vi "SpawnMediator.vi"(8 "Components":T1[](array[typedef]), 9 "Persistent":T1[](array[typedef]), 10 "MediatorAlias":string, 11 "Mediator":refnum<class "Actor.lvclass">) -> ()   [LabVIEW 2020, in "jettl.lvlib"]
uses:
  jettl.lvlib
  Message/Message.lvclass
  Base/Actor/Actor.lvclass
  C:/jettl-harness/repos/jettl/src/jettl/jettl/Base/Actor/Actor.lvclass
  C:/jettl-harness/repos/jettl/src/jettl/jettl/Actor/Actor.lvclass
  Actor/Actor.lvclass
  LifecycleEnum.ctl
  MessageCluster.ctl
  ActorTypeEnum.ctl
  MessageSet.ctl
  TellComponentMessageSetMap.ctl
  MessagesCluster.ctl
  ActorCluster.ctl
  PostSetupCluster.ctl
  SpawnComponent.vi
  MainCluster.ctl
  Base/Base.lvlib
  TellOriginEnum.ctl
  MetadataCluster.ctl
  ActorMap.ctl
  CustomMetadata/CustomMetadata.lvclass
panel:
  in  "Component":refnum<class "Actor.lvclass">
  in  "Actor in 2":refnum<class "Actor.lvclass">
  in  "Actors 2":refnum<class "Actor.lvclass">[](array[class])
  out "Actor out 2":refnum<class "Actor.lvclass">
  out "Actor out":refnum<class "Actor.lvclass">
  in  "Actor in":refnum<class "Actor.lvclass">
  in  "Actors":refnum<class "Actor.lvclass">[](array[class])
  in  "ActorAlias":string
  in  "Error in 2":errorcluster
  out "Error out 2":errorcluster
  in  "Teller 2":T2 {"AbsoluteTime" format="%<%x %.3X>T"}
  out "ConcreteActor 4":refnum<class "Actor.lvclass">
  in  "ConcreteActor 3":refnum<class "Actor.lvclass">
  in  "Error in":errorcluster
  out "Error out":errorcluster
  in  "Error":errorcluster
  in  "Teller":T2 {"AbsoluteTime" format="%<%x %.3X>T"}
  in  "Actor 2":refnum<class "Actor.lvclass">
  out "ConcreteActor":refnum<class "Actor.lvclass">
  in  "ConcreteActor 2":refnum<class "Actor.lvclass">
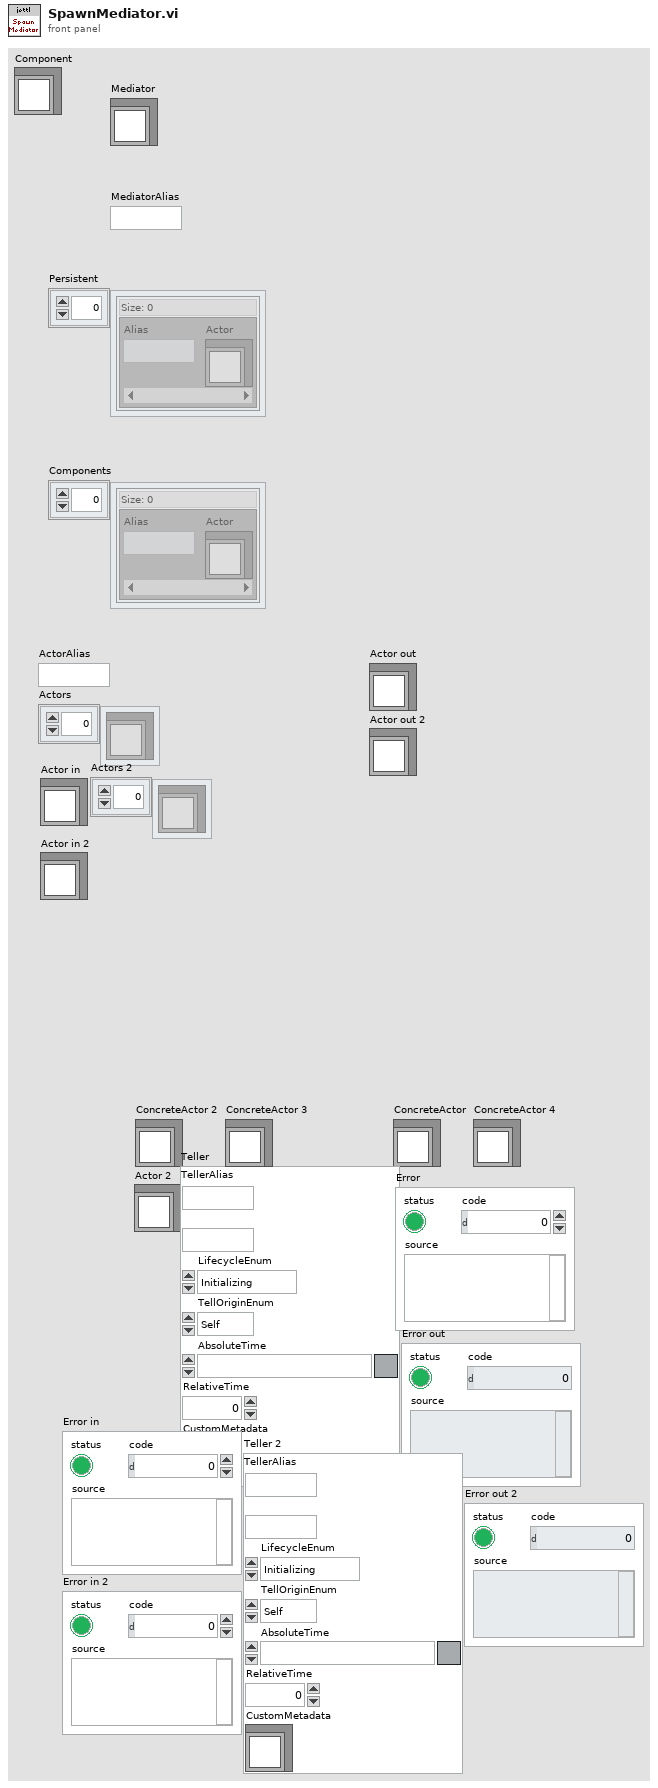
[diagram p1: front panel]
types:
  T1 = typedef "jettl.lvlib/ActorMap.ctl" = map{string, refnum<class "Actor.lvclass">}
  T2 = typedef "jettl.lvlib/MetadataCluster.ctl" = cluster{"TellerAlias":string, "ListenerAlias":string, "LifecycleEnum":T3, "TellOriginEnum":T4, "AbsoluteTime":timestamp, "RelativeTime":dbl, "CustomMetadata":refnum<class "CustomMetadata.lvclass">}
  T3 = typedef "jettl.lvlib/LifecycleEnum.ctl" = enum16{"Initializing", "SettingUp", "Starting", "Running", "Stopping", "TearingDown", "Terminated"}
  T4 = typedef "jettl.lvlib/TellOriginEnum.ctl" = enum16{"Self", "Mediator", "Component"}
  T5 = typedef "jettl.lvlib/MainCluster.ctl" = cluster{"SetupClusterQueue":refnum<queue>, "BeginSetupQueue":refnum<queue>, "SetupErrorQueue":refnum<queue>, "BeginStartQueue":refnum<queue>}
  T6 = typedef "jettl.lvlib/PostSetupCluster.ctl" = cluster{"VIRef":refnum<vi>, "Error":errorcluster}
  T7 = typedef "jettl.lvlib/ActorCluster.ctl" = cluster{"MessagesCluster":T8, "Alias":string, "ActorTypeEnum":T11, "MessageClusterDVREvent":refnum<user-event>, "EventRegistrationRef":refnum<event-registration>, "VIRef":refnum<vi>}
  T8 = typedef "jettl.lvlib/MessagesCluster.ctl" = cluster{"ListenMessageSet":T9, "TellSelfMessageSet":T9, "TellMediatorMessageSet":T9, "TellComponentMessageSetMap":T10}
  T9 = typedef "jettl.lvlib/MessageSet.ctl" = set{refnum<class "Message.lvclass">}
  T10 = typedef "jettl.lvlib/TellComponentMessageSetMap.ctl" = map{string, T9}
  T11 = typedef "jettl.lvlib/ActorTypeEnum.ctl" = enum16{"Mediator", "Component"}
  T12 = typedef "jettl.lvlib/BaseCluster.ctl" = cluster{"LifecycleEnum":T3, "MainCluster":T5, "SelfActorCluster":T7, "MediatorActorCluster":T7, "ComponentActorClusterMap":T13}
  T13 = typedef "jettl.lvlib/ComponentActorClusterMap.ctl" = map{string, T7}
  T14 = typedef "jettl.lvlib/AliasTellComponent.ctl" = map{string, T15}
  T15 = typedef "jettl.lvlib/Actor.ctl" = cluster{"Messages":T16, "ActorAlias":string, "ActorType":T18, "Transport":refnum<user-event>, "EventRegistrationRef":refnum<event-registration>, "VIRef":refnum<vi>}
  T16 = typedef "jettl.lvlib/Messages.ctl" = cluster{"Listen":T9, "TellSelf":T9, "TellMediator":T9, "TellComponentMap":T17}
  T17 = typedef "jettl.lvlib/TellComponent.ctl" = map{string, T9}
  T18 = typedef "jettl.lvlib/ActorType.ctl" = enum16{"Mediator", "Component"}
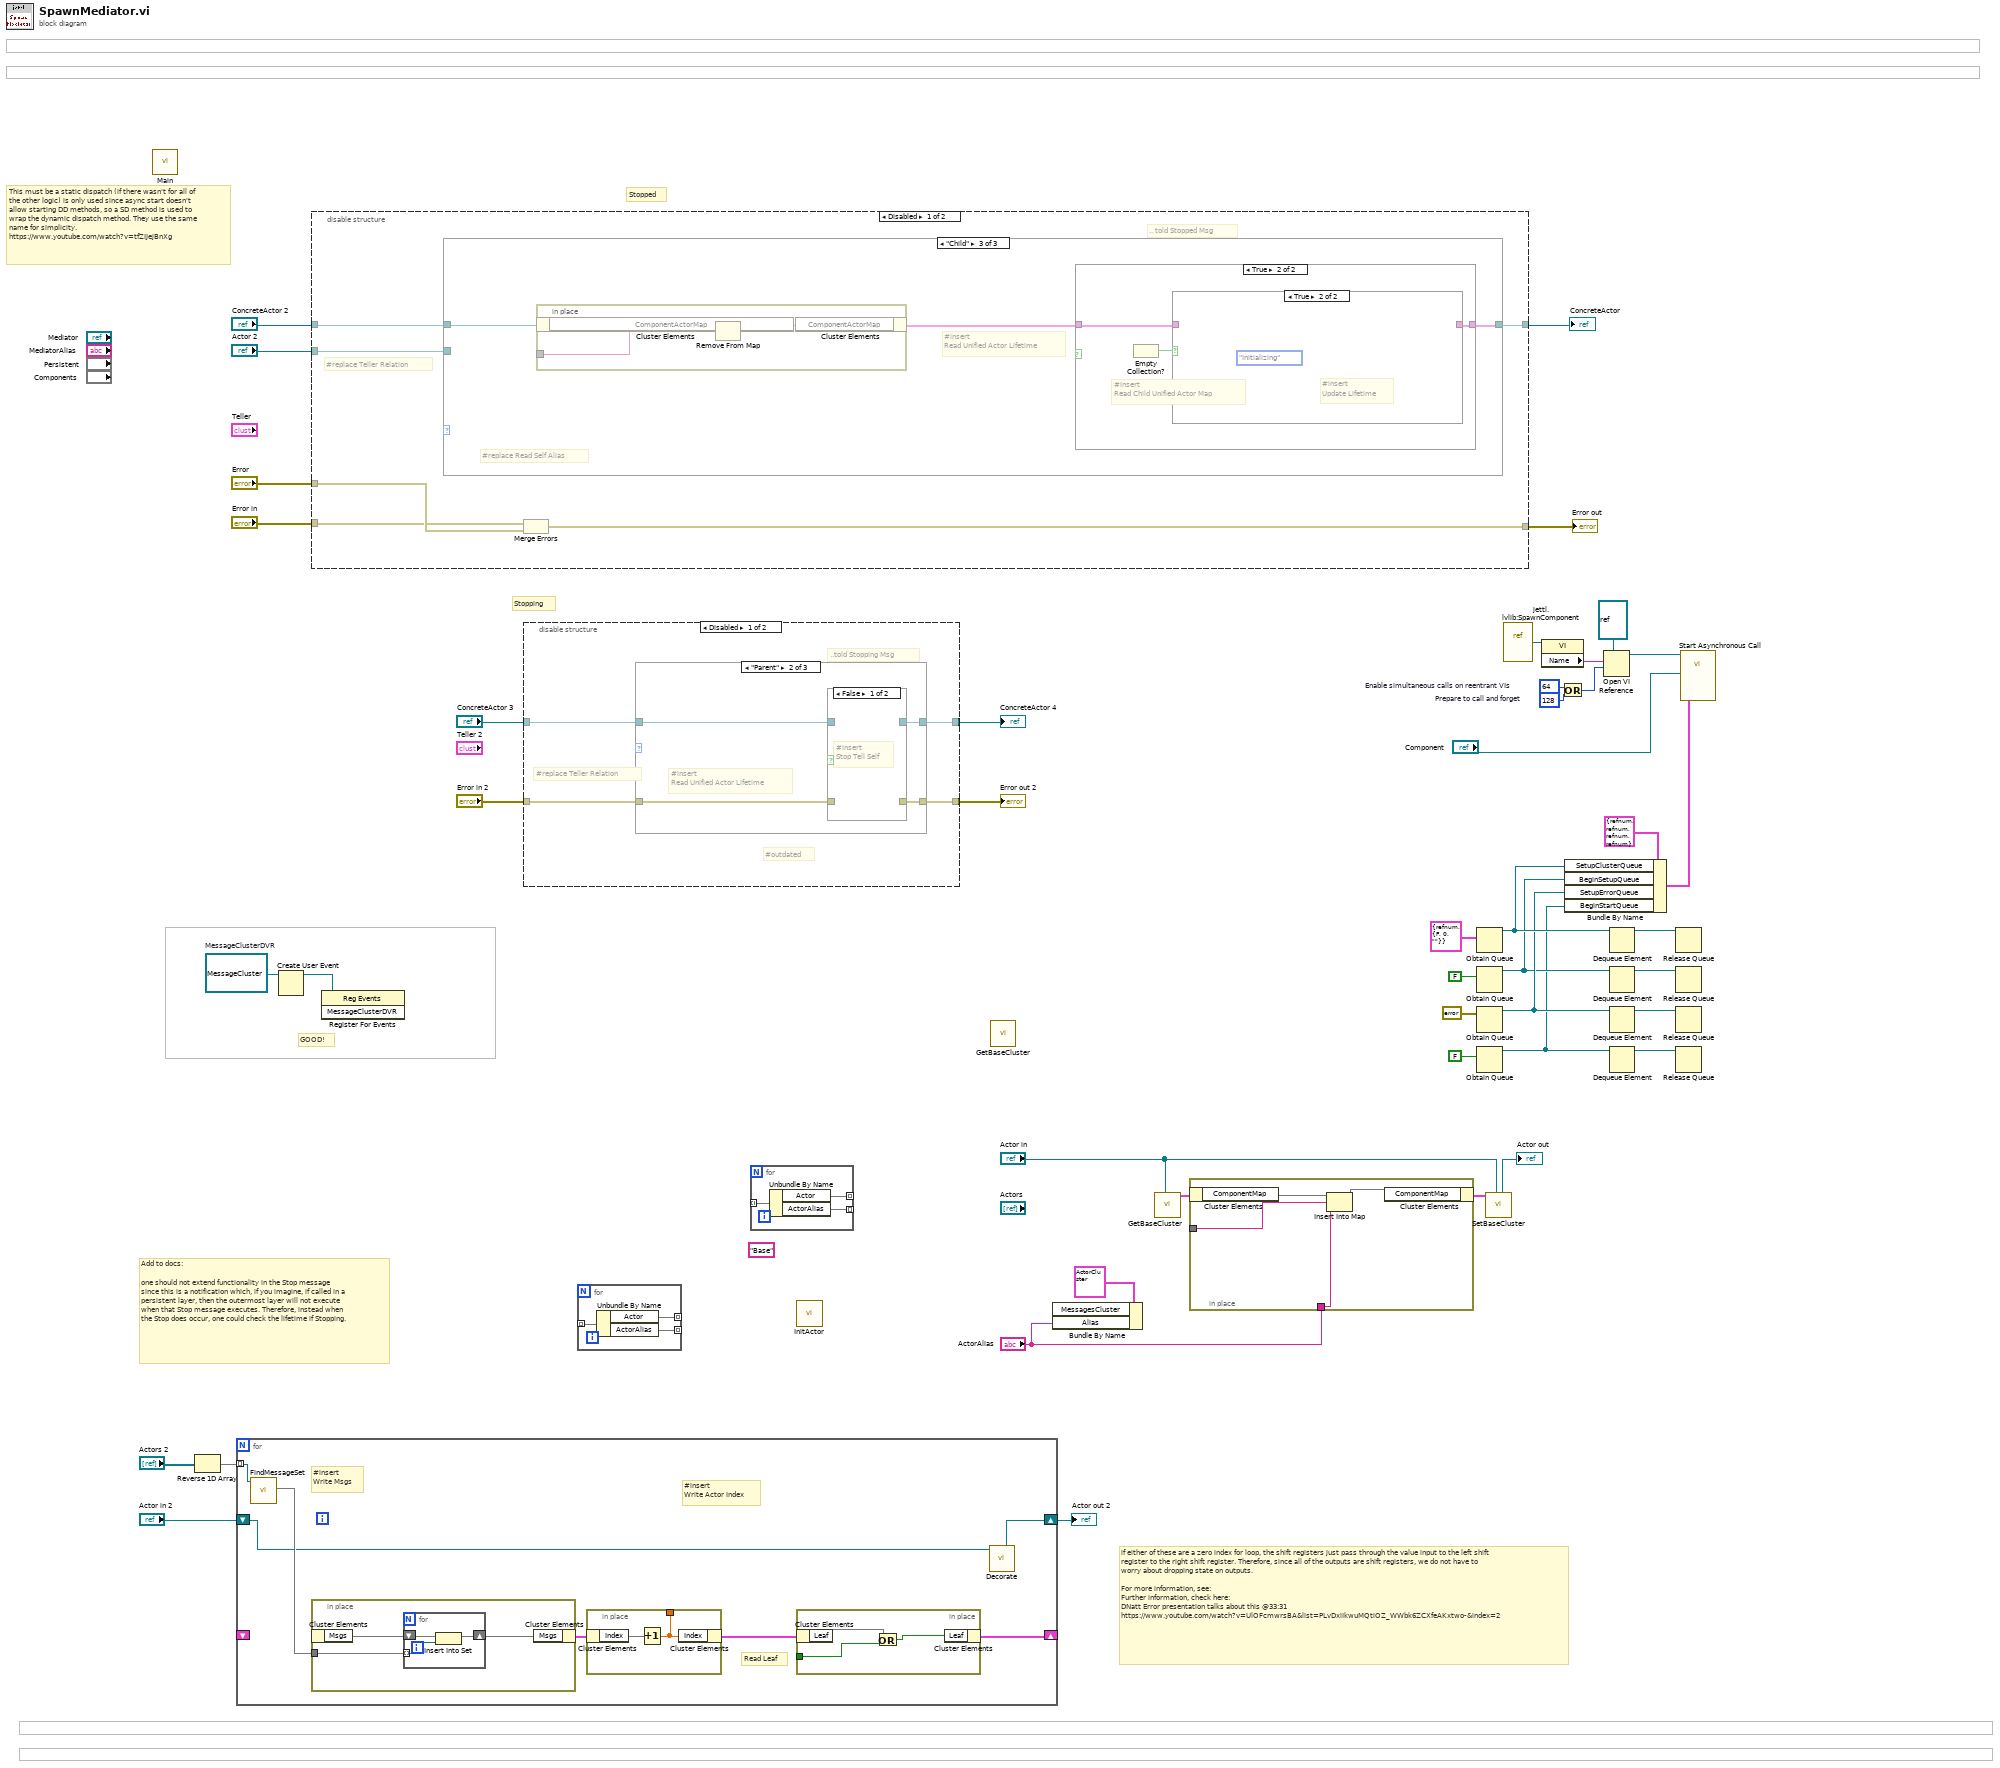
[diagram p0: block diagram]
diagram:
  w3 = refnum<data-value> refnum  # MessageClusterDVR
  w10 = 64  # Enable simultaneous calls on reentrant VIs
  w11 = 128  # Prepare to call and forget
  (unwired) "Base"
  # "GOOD!"
  # "if either of these are a zero index for loop, the shift registers just pass through the value input to the left shift register to the right shift register. Therefore, since all of the outputs are shift registers, we do not have to worry about dropping state on outputs.\n\nFor more information, see:\nFurther information, check here:\nDNatt Error presentation talks about this @33:31\nhttps://www.youtube.com/watch?v=UlOFcmwrsBA&list=PLvDxiIkwuMQtiOZ_WWbk6ZCXfeAKxtwo-&index=2"
  # "Add to docs:\n\none should not extend functionality in the Stop message since this is a notification which, if you imagine, if called in a persistent layer, then the outermost layer will not execute when that Stop message executes. Therefore, instead when the Stop does occur, one could check the lifetime if Stopping."
  # "Stopped"
  # "Stopping"
  # "This must be a static dispatch (if there wasn't for all of the other logic) is only used since async start doesn't allow starting DD methods, so a SD method is used to wrap the dynamic dispatch method. They use the same name for simplicity.\nhttps://www.youtube.com/watch?v=tfZIJejBnXg"
  n1 = call-dynamic "Main.vi"() -> ()  [unwired: 12 in]
  n2 = Reverse 1D Array(array="Actors 2") -> (reversed array=w33:refnum<class "Actor.lvclass">[])
  n3 = for {
    tunnel: w33 -> [w56] mode=indexing
    shift-right: [w51] -> w32
    shift-left: "Actor in 2" -> [w49]
    shift-right: [w57] -> w29
    shift-left: _ -> [_]
    # "#insert\nWrite Actor Index"
    # "#insert\nWrite Msgs"
    # "Read Leaf"
    n4 = call-dynamic "FindMessageSet.vi"(11:w56) -> (2:w58)  [unwired: 9 in, 1 out]
    n5 = in-place {
      in-place-border: w58 -> [w66]
      n6 = in-place-cluster #1() -> ("Msgs"=w65)  [unwired: 1 in]
      n7 = for {
        shift-right: [w68] -> w64
        shift-left: w65 -> [w69]
        tunnel: w66 -> [w67] mode=indexing
        n8 = Insert Into Set(10:w67, 11:w69) -> (3:w68:set{refnum<class "Message.lvclass">})  [unwired: 1 out]
      }
      n9 = in-place-cluster #1("Msgs"=w64) -> (w54:cluster{})
    }
    n10 = in-place {
      in-place-border: [w62] -> w52
      n11 = in-place-cluster #2(w54) -> ("Index"=w63)
      n12 = Increment(x=w63) -> (x+1=w62:dbl)
      n13 = in-place-cluster #2("Index"=w62) -> (w53:cluster{})
    }
    n14 = in-place {
      in-place-border: [w59] -> w55
      n15 = in-place-cluster #3(w53) -> ("Leaf"=w61)
      n16 = Or(x=w61, y=w59) -> (x .or. y?=w60:bool)
      n17 = in-place-cluster #3("Leaf"=w60) -> (w57:cluster{})
    }
    n18 = call-dynamic "Decorate.vi"("Actor"=w49) -> (5:"Actor"=w51:refnum<class "Actor.lvclass">, 7:"Actor"=w50:refnum<class "Actor.lvclass">)  [unwired: 9 in]
  }
  "Actor out 2" <- w32
  n19 = Create User Event(user event datatype=w3) -> (user event=w2:refnum<user-event>)  [unwired: 1 in, 1 out]
  n20 = disable-structure shown="Disabled" {
    disable-tunnel: [w75 w93] -> w48
    disable-tunnel: "ConcreteActor 2" -> [w74 w93]
    disable-tunnel: "Actor 2" -> [w73 _]
    disable-tunnel: "Error" -> [w72 _]
    disable-tunnel: "Error in" -> [w71 w94]
    disable-tunnel: [w70 w94] -> w43
    frame Disabled {
      # "#replace Teller Relation"
      # ".. told Stopped Msg"
      n21 = case shown="\"Child\"" {
        selector: _ -> [_ _ _]
        tunnel: w74 -> [w76 w77 w79]
        tunnel: [w76 w77 w81] -> w75
        tunnel: w73 -> [_ _ w80]
        frame "Self" {
          # "Case will not fundamentally execute"
        }
        frame "Parent" {
          # "Case will not fundamentally execute"
        }
        frame "Child" {
          # "#insert\nRead Unified Actor Lifetime"
          # "#replace Read Self Alias"
          n22 = in-place {
            in-place-border: [w84] -> _
            n23 = in-place-cluster #4(w79) -> ("ComponentActorMap"=w83)
            n24 = Remove From Map(11:w83) -> (3:w82:map{string, i32}, 10:w84:string)  [unwired: 2 out]
            n25 = in-place-cluster #4("ComponentActorMap"=w82) -> (w78:cluster{})
          }
          n26 = case shown="True" {
            selector: _ -> [_ _]
            tunnel: w78 -> [w85 w86]
            tunnel: [w85 w88] -> w81
            frame False {
            }
            frame True {
              # "#insert\nRead Child Unified Actor Map"
              n27 = Empty Collection?() -> (0:w87:bool)  [unwired: 1 in]
              n28 = case shown="True" w87 {
                tunnel: [w89 w90] -> w88
                tunnel: w86 -> [w89 w91]
                frame False {
                }
                frame True {
                  w92 = LifecycleEnum."Initializing" ("Lifetime")
                  # "#insert\nUpdate Lifetime"
                }
              }
            }
          }
        }
      }
      n29 = Merge Errors(w71, w72) -> (w70:errorcluster)
    }
    frame Enabled {
    }
  }
  "ConcreteActor" <- w48
  "Error out" <- w43
  n30 = register-events(w2) -> (reference out=w1:refnum<event-registration>)  [unwired: 2 in, 1 out]
  n31 = disable-structure shown="Disabled" {
    disable-tunnel: "ConcreteActor 3" -> [w98 w113]
    disable-tunnel: [w97 w113] -> w41
    disable-tunnel: "Error in 2" -> [w96 w112]
    disable-tunnel: [w95 w112] -> w39
    frame Disabled {
      # "#outdated"
      # "#replace Teller Relation"
      # "..told Stopping Msg"
      n32 = case shown="\"Parent\"" {
        selector: _ -> [_ _ _]
        tunnel: w98 -> [w100 w101 w111]
        tunnel: [w100 w104 w111] -> w97
        tunnel: w96 -> [w99 w103 w110]
        tunnel: [w99 w102 w110] -> w95
        frame "Self" {
          # "Case will not fundamentally execute"
        }
        frame "Parent" {
          # "#insert\nRead Unified Actor Lifetime"
          n33 = case shown="False" {
            selector: _ -> [_ _]
            tunnel: [w107 w109] -> w104
            tunnel: w103 -> [w106 w108]
            tunnel: [_ w108] -> w102
            tunnel: w101 -> [w105 w109]
            frame False {
              # "#insert\nStop Tell Self"
            }
            frame True {
            }
          }
        }
        frame "Child" {
          # "Case will not fundamentally execute"
        }
      }
    }
    frame Enabled {
    }
  }
  "ConcreteActor 4" <- w41
  "Error out 2" <- w39
  n34 = for {
    tunnel: [w116] -> _ mode=indexing
    tunnel: [w115] -> _ mode=indexing
    tunnel: _ -> [w114] mode=indexing
    n35 = Unbundle By Name(w114) -> ("Actor"=w116, "ActorAlias"=w115)
  }
  n36 = for {
    tunnel: [w119] -> _ mode=indexing
    tunnel: [w118] -> _ mode=indexing
    tunnel: _ -> [w117] mode=indexing
    n37 = Unbundle By Name(w117) -> ("Actor"=w119, "ActorAlias"=w118)
  }
  n38 = call "InitActor.vi"() -> ()  [unwired: 11 in, 1 out]
  n39 = call-dynamic "GetBaseCluster.vi"() -> ()  [unwired: 11 in, 1 out]
  n40 = Bundle By Name(cluster=T7 {"MessagesCluster"={"ListenMessageSet"={}, "TellSelfMessageSet"={}, "TellMediatorMessageSet"={}, "TellComponentMessageSetMap"={}}, "Alias"="", "ActorTypeEnum"=enum."Mediator", "MessageClusterDVREvent"=refnum, "EventRegistrationRef"=refnum, "VIRef"=refnum} ("Attributes"), "Alias"="ActorAlias") -> (w34:T7)  [unwired: 1 in]
  n41 = call-dynamic "GetBaseCluster.vi"("Actor"="Actor in") -> ("BaseCluster"=w17:T12)  [unwired: 10 in]
  n42 = in-place {
    in-place-border: "ActorAlias" -> [w123]
    in-place-border: [w122] -> w15
    n43 = in-place-cluster #5(w17) -> ("ComponentMap"=w121:T14)
    n44 = Insert Into Map(map in=w121, value=w123) -> (key=w122:string, map out=w120:T14)  [unwired: 2 out]
    n45 = in-place-cluster #5("ComponentMap"=w120) -> (w16:T12)
  }
  n46 = Obtain Queue(element data type=T6 {"VIRef"=refnum, "Error"={"status"=FALSE, "code"=0, "source"=""}} ("PreSetup")) -> (queue out=w25:refnum<queue>)  [unwired: 4 in, 2 out]
  n47 = Obtain Queue(element data type=FALSE) -> (queue out=w20:refnum<queue>)  [unwired: 4 in, 2 out]
  n48 = Obtain Queue(element data type=errorcluster {"status"=FALSE, "code"=0, "source"=""} ("Error")) -> (queue out=w21:refnum<queue>)  [unwired: 4 in, 2 out]
  n49 = Obtain Queue(element data type=FALSE) -> (queue out=w19:refnum<queue>)  [unwired: 4 in, 2 out]
  n50 = call-dynamic "SetBaseCluster.vi"("Actor"="Actor in", "BaseCluster"=w16) -> ("Actor"=→"Actor out":refnum<class "Actor.lvclass">)  [unwired: 9 in]
  n51 = vi-ref "jettl.lvlib:SpawnComponent.vi"() -> (w13:refnum<vi>)
  n52 = property class="VI"(reference=w13) -> ("Name"=w14:string)  [unwired: 1 in, 2 out]
  n53 = Or(x=w10, y=w11) -> (x .or. y?=w9:i32)
  n54 = Bundle By Name(cluster=T5 {"SetupClusterQueue"=refnum, "BeginSetupQueue"=refnum, "SetupErrorQueue"=refnum, "BeginStartQueue"=refnum} ("MainCluster"), "SetupClusterQueue"=w25, "BeginSetupQueue"=w20, "SetupErrorQueue"=w21, "BeginStartQueue"=w19) -> (w6:T5)
  n55 = Open VI Reference(type specifier VI Refnum (for type only)=refnum<vi> refnum, vi path=w14, options=w9) -> (vi reference=w8:refnum<vi>)  [unwired: 3 in, 1 out]
  n56 = Dequeue Element(queue=w25) -> (queue out=w26:refnum<queue>)  [unwired: 2 in, 3 out]
  n57 = Dequeue Element(queue=w20) -> (queue out=w28:refnum<queue>)  [unwired: 2 in, 3 out]
  n58 = Dequeue Element(queue=w21) -> (queue out=w24:refnum<queue>)  [unwired: 2 in, 3 out]
  n59 = Dequeue Element(queue=w19) -> (queue out=w5:refnum<queue>)  [unwired: 2 in, 3 out]
  n60 = Release Queue(queue=w26) -> ()  [unwired: 2 in, 3 out]
  n61 = Release Queue(queue=w28) -> ()  [unwired: 2 in, 3 out]
  n62 = Release Queue(queue=w24) -> ()  [unwired: 2 in, 3 out]
  n63 = Release Queue(queue=w5) -> ()  [unwired: 2 in, 3 out]
  n64 = call-by-ref "Start Asynchronous Call"(reference=w8, "MainCluster"=w6, "Component"="Component") -> ()  [unwired: 11 in, 2 out]
